vi "ReSortPoints.vi"(8 "error in (no error)":errorcluster, 10 "DutyCluster":T1 {"Iteration" items=["first iteration", "second iteration"]}, 11 "XYZ Point coordinates (pixels)":dbl[][](array[numeric])) -> (0 "error out":errorcluster, 3 "Point coordinates resorte (pixels)":dbl[][](array[numeric]))   [LabVIEW 2010]
uses:
  TypeDefs/DutyCluster.ctl
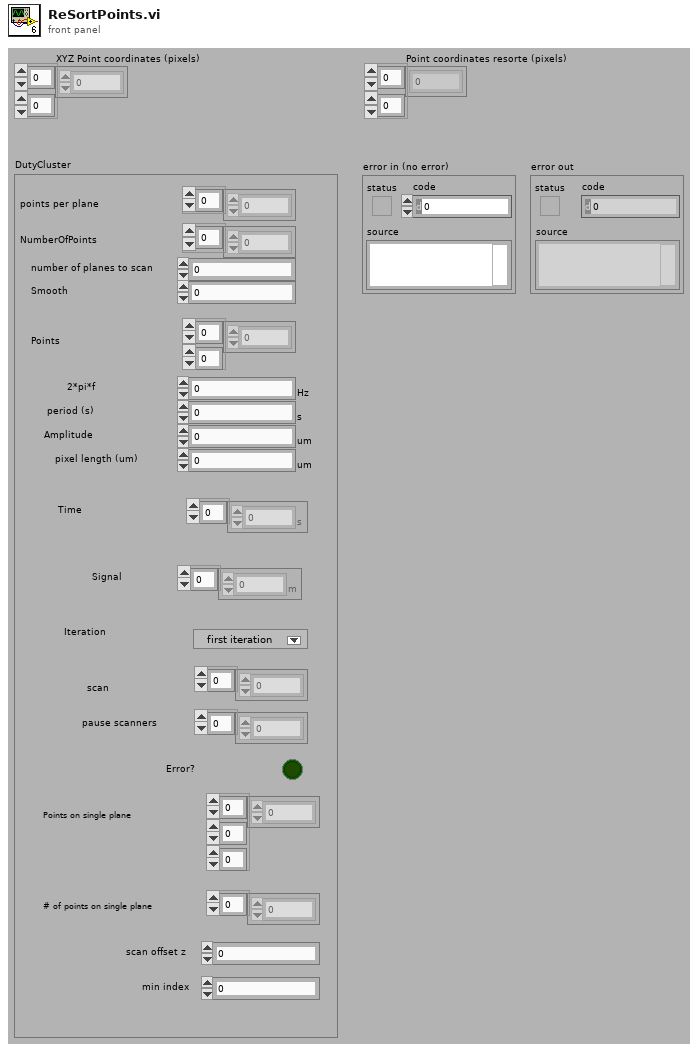
[diagram p1: front panel]
types:
  T1 = typedef "DutyCluster.ctl" = cluster{"points per plane":i32[], "NumberOfPoints":i32[], "number of planes to scan":i32, "Smooth":i32, "Points":dbl[][], "2*pi*f":dbl[unit], "period (s)":dbl[unit], "Amplitude":dbl[unit], "pixel length (um)":dbl[unit], "Time":dbl[unit][], "Signal":dbl[unit][], "Iteration":u16, "scan":i32[], "pause scanners":i32[], "Error?":bool, "Points on single plane":dbl[][][], "# of points on single plane":i32[], "scan offset z":i32, "min index":i32}
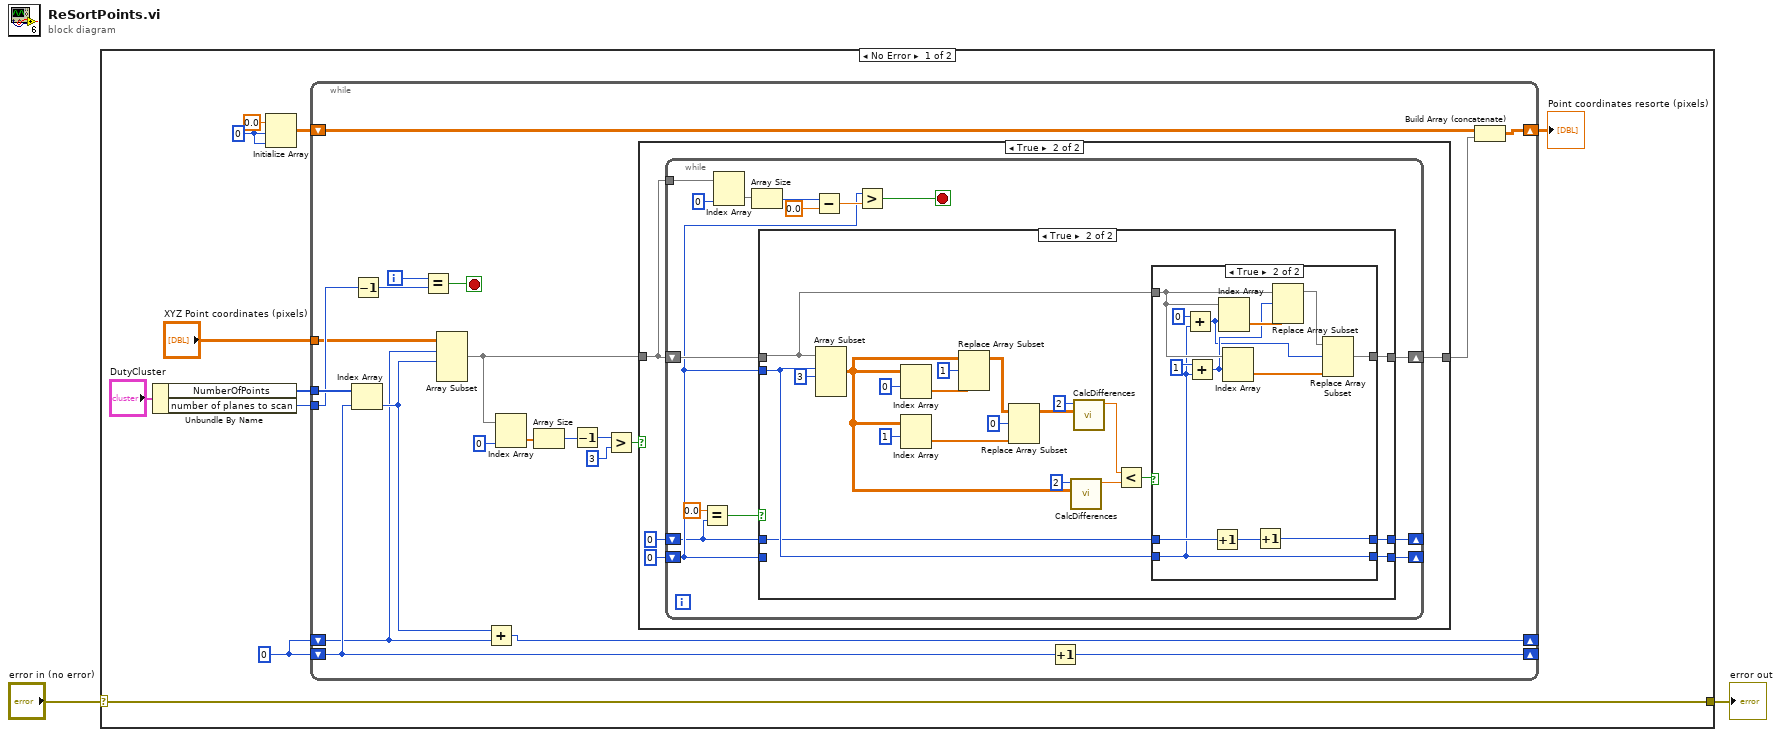
[diagram p0: block diagram]
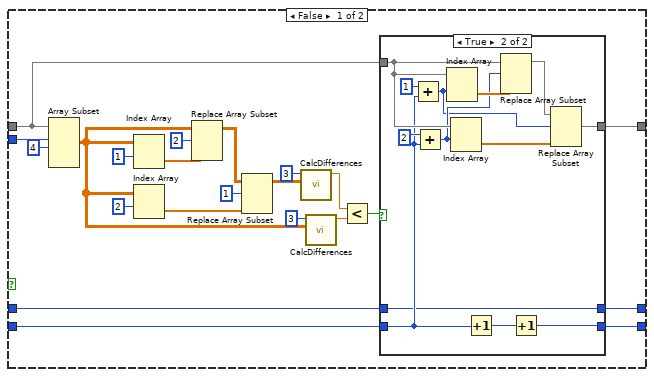
[diagram p3: hidden frame]
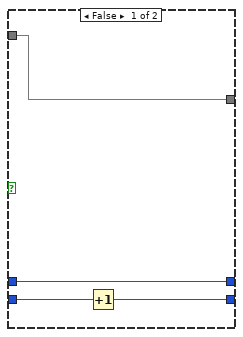
[diagram p4: hidden frame]
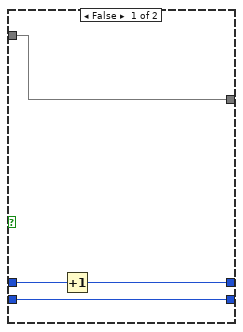
[diagram p5: hidden frame]
diagram:
  n1 = case shown="No Error" "error in (no error)" {
    selector: "error in (no error)" -> [w8 w131]
    tunnel: [w8 w131] -> w1
    frame No Error {
      w3 = 0 ("dimension size")
      w4 = 0 ("index (page)")
      n2 = Unbundle By Name("DutyCluster") -> ("NumberOfPoints"=w6:i32[], "number of planes to scan"=w5:i32)
      n3 = Initialize Array(0.0 ("element"), w3, w3) -> (w11:dbl[][])
      n4 = while {
        tunnel: "XYZ Point coordinates (pixels)" -> [w14]
        shift-right: [w31] -> _
        shift-left: w4 -> [w15]
        shift-right: [w30] -> w9
        shift-left: w11 -> [w29]
        tunnel: w6 -> [w27]
        tunnel: w5 -> [w18]
        shift-right: [w16] -> _
        shift-left: w4 -> [w13]
        i -> [w33]
        stop <- w32 stop-if-true
        n5 = Index Array(array=w27, index=w15) -> (element=w17:i32)
        n6 = Decrement(x=w18) -> (x-1=w28:i32)
        n7 = Equal?(x=w33, y=w28) -> (x = y?=w32:bool)
        n8 = Array Subset(array=w14, index (row)=w13, length (row)=w17) -> (w23:dbl[][])  [unwired: 2 in]
        n9 = Add(x=w17, y=w13) -> (x+y=w16:i32)
        n10 = Index Array(array=w23, index (col)=0 ("index (row)")) -> (element=w25:dbl[])  [unwired: 1 in]
        n11 = Array Size(array=w25) -> (size(s)=w21:i32)
        n12 = Decrement(x=w21) -> (x-1=w20:i32)
        n13 = Greater?(x=w20, y=3) -> (0:w24:bool)
        n14 = case shown="True" w24 {
          tunnel: [w34 w37] -> w19
          tunnel: w23 -> [w34 w36]
          frame False {
          }
          frame True {
            n15 = while {
              shift-right: [w51] -> _
              shift-left: 0 ("length") -> [w42]
              shift-right: [w52] -> w37
              shift-left: w36 -> [w53]
              tunnel: w36 -> [w45]
              shift-right: [w43] -> _
              shift-left: 0 ("length") -> [w41]
              stop <- w46 stop-if-true
              n16 = Equal?(x=0.0 ("y"), y=w41) -> (x = y?=w39:bool)
              n17 = Index Array(array=w45, index (col)=0 ("disabled index (col)")) -> (element=w48:dbl[])  [unwired: 1 in]
              n18 = Array Size(array=w48) -> (size(s)=w50:i32)
              n19 = case shown="True" w39 {
                tunnel: w53 -> [w68 w104]
                tunnel: [w66 w102] -> w52
                tunnel: [w64 w101] -> w51
                tunnel: w42 -> [w63 w103]
                tunnel: w41 -> [w62 w100]
                tunnel: [w61 w99] -> w43
                tunnel: w42 -> [w60 _]
                frame False {
                  n20 = Array Subset(array=w68, index (row)=w63, length (row)=4 ("length")) -> (w55:dbl[][])  [unwired: 2 in]
                  n21 = Index Array(array=w55, index (row)=1) -> (element=w69:dbl[])  [unwired: 1 in]
                  n22 = Index Array(array=w55, index (row)=2) -> (element=w70:dbl[])  [unwired: 1 in]
                  n23 = Replace Array Subset(array=w55, new element=w69, index (row)=2) -> (w67:dbl[][])  [unwired: 1 in]
                  n24 = Replace Array Subset(array=w67, new element=w70, index (row)=1) -> (w58:dbl[][])  [unwired: 1 in]
                  n25 = call "CalcDifferences.vi"("PointsIn (pixels)"=w58, "Iterations"=3) -> ("Differences"=w57:dbl)  [unwired: 8 in, 1 out]
                  n26 = call "CalcDifferences.vi"("PointsIn (pixels)"=w55, "Iterations"=3) -> ("Differences"=w54:dbl)  [unwired: 8 in, 1 out]
                  n27 = Less?(x=w57, y=w54) -> (x < y?=w65:bool)
                  n28 = case shown="True" w65 {
                    tunnel: w68 -> [w79 w90]
                    tunnel: [w79 w88] -> w66
                    tunnel: w60 -> [w78 w83]
                    tunnel: [w77 w80] -> w64
                    tunnel: w62 -> [w76 w82]
                    tunnel: [w76 w82] -> w61
                    frame False {
                      n29 = Increment(x=w78) -> (x+1=w77:i32)
                    }
                    frame True {
                      n30 = Add(x=1 ("index (row)"), y=w83) -> (x+y=w84:i32)
                      n31 = Add(x=2 ("index (row)"), y=w83) -> (x+y=w85:i32)
                      n32 = Index Array(array=w90, index (row)=w84) -> (element=w91:dbl[])  [unwired: 1 in]
                      n33 = Index Array(array=w90, index (row)=w85) -> (element=w92:dbl[])  [unwired: 1 in]
                      n34 = Increment(x=w83) -> (x+1=w81:i32)
                      n35 = Replace Array Subset(array=w90, new element=w91, index (row)=w85) -> (w89:dbl[][])  [unwired: 1 in]
                      n36 = Increment(x=w81) -> (x+1=w80:i32)
                      n37 = Replace Array Subset(array=w89, new element=w92, index (row)=w84) -> (w88:dbl[][])  [unwired: 1 in]
                    }
                  }
                }
                frame True {
                  n38 = Array Subset(array=w104, index (row)=w103, length (row)=3 ("length")) -> (w94:dbl[][])  [unwired: 2 in]
                  n39 = Index Array(array=w94, index (row)=0) -> (element=w107:dbl[])  [unwired: 1 in]
                  n40 = Index Array(array=w94, index (row)=1) -> (element=w108:dbl[])  [unwired: 1 in]
                  n41 = Replace Array Subset(array=w94, new element=w107, index (row)=1) -> (w106:dbl[][])  [unwired: 1 in]
                  n42 = Replace Array Subset(array=w106, new element=w108, index (row)=0) -> (w97:dbl[][])  [unwired: 1 in]
                  n43 = call "CalcDifferences.vi"("PointsIn (pixels)"=w94, "Iterations"=2) -> ("Differences"=w93:dbl)  [unwired: 8 in, 1 out]
                  n44 = call "CalcDifferences.vi"("PointsIn (pixels)"=w97, "Iterations"=2) -> ("Differences"=w96:dbl)  [unwired: 8 in, 1 out]
                  n45 = Less?(x=w96, y=w93) -> (x < y?=w105:bool)
                  n46 = case shown="True" w105 {
                    tunnel: w104 -> [w117 w128]
                    tunnel: [w117 w126] -> w102
                    tunnel: w103 -> [w114 w120]
                    tunnel: [w114 w120] -> w101
                    tunnel: w100 -> [w116 w121]
                    tunnel: [w115 w118] -> w99
                    frame False {
                      n47 = Increment(x=w116) -> (x+1=w115:i32)
                    }
                    frame True {
                      n48 = Add(x=0 ("index (row)"), y=w120) -> (x+y=w122:i32)
                      n49 = Add(x=1 ("index (row)"), y=w120) -> (x+y=w123:i32)
                      n50 = Increment(x=w121) -> (x+1=w119:i32)
                      n51 = Index Array(array=w128, index (row)=w122) -> (element=w129:dbl[])  [unwired: 1 in]
                      n52 = Index Array(array=w128, index (row)=w123) -> (element=w130:dbl[])  [unwired: 1 in]
                      n53 = Increment(x=w119) -> (x+1=w118:i32)
                      n54 = Replace Array Subset(array=w128, new element=w129, index (row)=w123) -> (w127:dbl[][])  [unwired: 1 in]
                      n55 = Replace Array Subset(array=w127, new element=w130, index (row)=w122) -> (w126:dbl[][])  [unwired: 1 in]
                    }
                  }
                }
              }
              n56 = Subtract(x=w50, y=0.0) -> (x-y=w44:dbl)
              n57 = Greater?(x=w42, y=w44) -> (0:w46:bool)
            }
          }
        }
        n58 = Increment(x=w15) -> (x+1=w31:i32)
        n59 = Build Array (concatenate)(w29, w19) -> (w30:dbl[][])
      }
      "Point coordinates resorte (pixels)" <- w9
    }
    frame Error {
    }
  }
  "error out" <- w1
